vi "Obtain Msg Q DVR.vi"(10 "Msg Q DVR Alias":string) -> (0 "error out":errorcluster, 2 "Msg Q DVR":refnum<data-value>)   [LabVIEW 2021, in "LVCAM.lvlib" / "Self Actor.lvclass"]
uses:
  Self Actor.lvclass
  Msg/Msg.lvclass
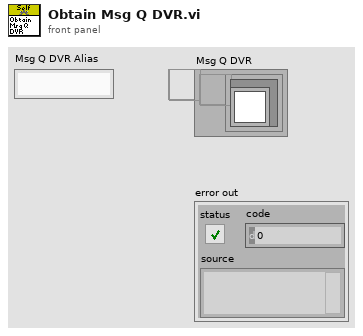
[diagram p1: front panel]
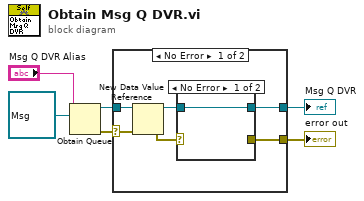
[diagram p0: block diagram]
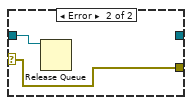
[diagram p3: hidden frame]
diagram:
  n1 = Obtain Queue(name (unnamed)="Msg Q DVR Alias", element data type=refnum<class "Msg.lvclass"> refnum ("Artifex Actor Model.lvlib:Msg.lvclass")) -> (queue out=w3:refnum<queue>, error out=w6:errorcluster)  [unwired: 3 in, 1 out]
  n2 = case shown="No Error" w6 {
    selector: w6 -> [w12 w15]
    tunnel: w3 -> [w11 w16]
    tunnel: [w8 _] -> w2
    tunnel: [w9 w15] -> w1
    frame No Error {
      n3 = New Data Value Reference(data value=w11, error in=w12) -> (data value reference=w7:refnum<data-value>, error out=w10:errorcluster)
      n4 = case shown="No Error" w10 {
        selector: w10 -> [_ w14]
        tunnel: [_ w14] -> w9
        tunnel: [w13 _] -> w8
        tunnel: w7 -> [w13 _]
        frame No Error {
        }
        frame Error {
        }
      }
    }
    frame Error {
      n5 = Release Queue(queue=w16) -> ()  [unwired: 2 in, 3 out]
    }
  }
  "Msg Q DVR" <- w2
  "error out" <- w1
